vi "Multi-VI-Hacker.vi"() -> ()   [LabVIEW 2020, in "VI-Hacker.lvlib"]
uses:
  VI-Hacker.lvlib
panel:
  in  "Overwrite":bool
  out "Progress":dbl(slide) scale=0.0..100.0
  in  "Target Folder":path
  in  "Source Folder":path caption="(15 found)"
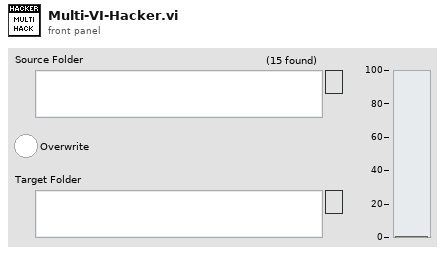
[diagram p1: front panel]
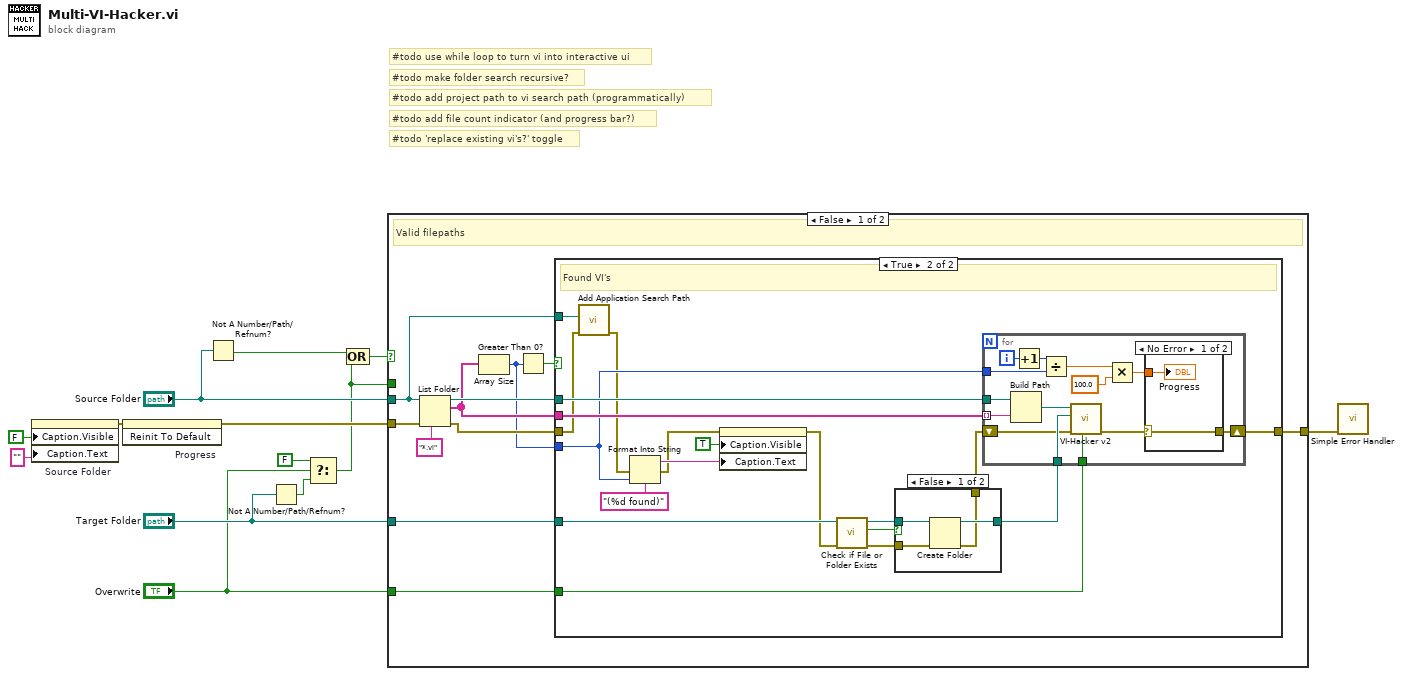
[diagram p0: block diagram]
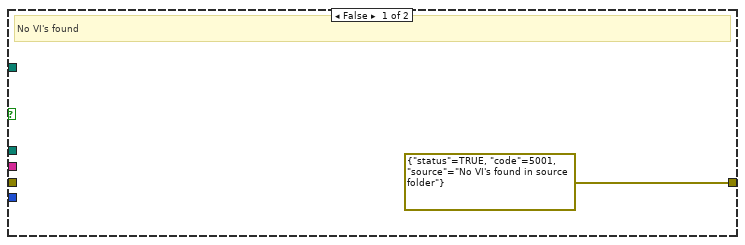
[diagram p2: hidden frame]
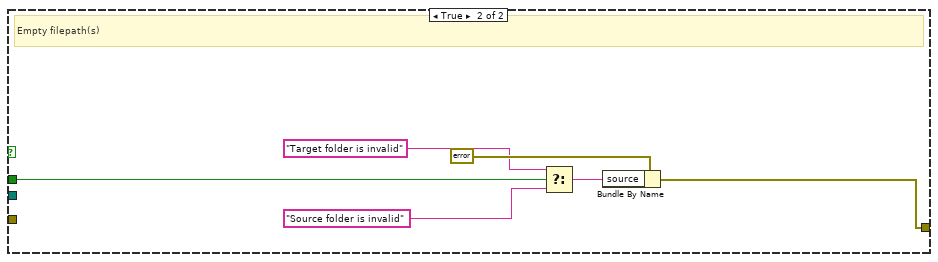
[diagram p5: hidden frame]
diagram:
  # "#todo use while loop to turn vi into interactive ui"
  # "#todo 'replace existing vi's?' toggle"
  # "#todo add file count indicator (and progress bar?)"
  # "#todo add project path to vi search path (programmatically)"
  # "#todo make folder search recursive?"
  n1 = property on="Source Folder" class="Path"("Caption.Visible"=FALSE ("Visible"), "Caption.Text"="") -> (error out=w8:errorcluster)  [unwired: 2 in, 1 out]
  n2 = invoke on="Progress" class="Slide (strict)" method="Reinit To Default"(error in=w8) -> (error out=w5:errorcluster)  [unwired: 2 in, 2 out]
  n3 = Not A Number/Path/Refnum?(number/path/refnum="Source Folder") -> (NaN/Path/Refnum?=w13:bool)
  n4 = Not A Number/Path/Refnum?(number/path/refnum="Target Folder") -> (NaN/Path/Refnum?=w4:bool)
  n5 = Select(t=FALSE, s="Overwrite", f=w4) -> (s? t:f=w3:bool)
  n6 = Compound Arithmetic op=OR(w13, w3) -> (w11:bool)
  n7 = case shown="False" w11 {
    tunnel: "Source Folder" -> [w16 _]
    tunnel: "Target Folder" -> [w20 _]
    tunnel: [w19 w68] -> w9
    tunnel: w3 -> [_ w72]
    tunnel: w5 -> [w15 _]
    tunnel: "Overwrite" -> [w14 _]
    frame False {
      # "Valid filepaths"
      n8 = List Folder(path=w16, pattern="*.vi", error in=w15) -> (path out=w23:path, filenames=w22:string[], error out=w18:errorcluster)  [unwired: 1 in, 1 out]
      n9 = Array Size(array=w22) -> (size(s)=w17:i32)
      n10 = Greater Than 0?(x=w17) -> (x > 0?=w21:bool)
      n11 = case shown="True" w21 {
        tunnel: w22 -> [_ w44]
        tunnel: w23 -> [_ w43]
        tunnel: w20 -> [_ w36]
        tunnel: [errorcluster {"status"=TRUE, "code"=5001, "source"="No VI's found in source folder"} ("error in (no error)") w42] -> w19
        tunnel: w18 -> [_ w37]
        tunnel: w17 -> [_ w30]
        tunnel: w16 -> [_ w38]
        tunnel: w14 -> [_ w26]
        frame False {
          # "No VI's found"
        }
        frame True {
          # "Found VI's"
          n12 = call "Add Application Search Path.vi"("error in"=w37, "New Search Path"=w38) -> ("error out"=w29:errorcluster)  [unwired: 6 in, 3 out]
          n13 = Format Into String(format string="(%d found)", error in=w29, w30) -> (resulting string=w31:string, error out=w28:errorcluster)  [unwired: 1 in]
          n14 = property on="Source Folder" class="Path"(error in=w28, "Caption.Visible"=TRUE, "Caption.Text"=w31) -> (error out=w32:errorcluster)  [unwired: 1 in, 1 out]
          n15 = call <vilib>:"Check if File or Folder Exists.vi"("error in (no error)"=w32, "path"=w36) -> ("error out"=w33:errorcluster, "file or folder exists?"=w34:bool, "dup path"=w35:path)  [unwired: 7 in]
          n16 = case shown="False" w34 {
            tunnel: [w48 w49] -> w41
            tunnel: [w47 w50] -> w40
            tunnel: w35 -> [w46 w49]
            tunnel: w33 -> [w45 w50]
            frame False {
              n17 = Create Folder(path (use dialog)=w46, error in=w45) -> (created path=w48:path, error out=w47:errorcluster)  [unwired: 1 in, 1 out]
            }
            frame True {
            }
          }
          n18 = for {
            tunnel: w43 -> [w64]
            tunnel: w44 -> [w63] mode=indexing
            tunnel: w41 -> [w61]
            shift-right: [w53] -> w42
            shift-left: w40 -> [w60]
            tunnel: w30 -> [w58]
            tunnel: w26 -> [w51]
            i -> [w59]
            n19 = Build Path(base path=w64, name or relative path=w63) -> (appended path=w62:path)
            n20 = Increment(x=w59) -> (x+1=w54:i32)
            n21 = Divide(x=w54, y=w58) -> (x/y=w57:dbl)
            n22 = call "VI-Hacker v2.vi"("Overwrite VI? (F)"=w51, "error in (no error)"=w60, "Target Folder"=w61, "VI Path"=w62) -> ("error out"=w52:errorcluster)  [unwired: 7 in]
            n23 = Multiply(x=w57, y=100.0) -> (x*y=w55:dbl)
            n24 = case shown="No Error" w52 {
              selector: w52 -> [w65 w67]
              tunnel: w55 -> [w66 _]
              tunnel: [w65 w67] -> w53
              frame No Error {
                "Progress" <- w66
              }
              frame Error {
              }
            }
          }
        }
      }
    }
    frame True {
      # "Empty filepath(s)"
      n25 = Select(t="Target folder is invalid" ("source"), s=w72, f="Source folder is invalid" ("source")) -> (s? t:f=w69:string)
      n26 = Bundle By Name(cluster=errorcluster {"status"=TRUE, "code"=5000, "source"="%s folder is invalid"} ("error in (no error)"), "source"=w69) -> (w68:errorcluster)
    }
  }
  n27 = call <vilib>:"Simple Error Handler.vi"("error in (no error)"=w9) -> ()  [unwired: 4 in, 5 out]
